vi "AutoGetRoutine.vi"(1 "Auto Routine":T6) -> (0 "Output Routine":T1[](array[typedef]))   [LabVIEW 2017]
uses:
  TypeDef/AutoRoutines.ctl
  TypeDef/AutoStep.ctl
  TypeDef/AutoWaypointType.ctl
  Pathfinder/Pathfinder-LabVIEW/Pathfinder-Lib/VIs/Waypoint.ctl
  Implements/Arm/TypeDefs/ArmTargetPosition.ctl
  Implements/TypeDefs/IntakeState.ctl
  Pathfinder/Pathfinder-LabVIEW/Pathfinder-Lib/Pathfinder.lvlib
panel:
  in  "Routines":T1[][](array[typedef])=[[{"Waypoint Type"=enum."Pathfinder Endpoint", "Waypoint"={"x"=19.5, "y"=160.0, "angle"=0.0}, "WaitTime (ms)"=0, "ArmPosition"=enum."Hold", "IntakeState"=enum."Stop", "Claw Open"=FALSE}, {"Waypoint Type"=enum."Pathfinder Endpoint", "Waypoint"={"x"=151.0, "y"=225.0, "angle"=0.0}, "WaitTime (ms)"=0, "ArmPosition"=enum."Switch", "IntakeState"=enum."Stop", "Claw Open"=FALSE}, {"Waypoint Type"=enum."Stationary", "Waypoint"={"x"=0.0, "y"=0.0, "angle"=0.0}, "WaitTime (ms)"=250, "ArmPosition"=enum."Switch", "IntakeState"=enum."Stop", "Claw Open"=TRUE}, {"Waypoint Type"=enum."Pathfinder Endpoint", "Waypoint"={"x"=0.0, "y"=0.0, "angle"=0.0}, "WaitTime (ms)"=0, "ArmPosition"=enum."Hold", "IntakeState"=enum."Stop", "Claw Open"=FALSE}, {"Waypoint Type"=enum."Pathfinder Endpoint", "Waypoint"={"x"=0.0, "y"=0.0, "angle"=0.0}, "WaitTime (ms)"=0, "ArmPosition"=enum."Hold", "IntakeState"=enum."Stop", "Claw Open"=FALSE}, {"Waypoint Type"=enum."Pathfinder Endpoint", "Waypoint"={"x"=0.0, "y"=0.0, "angle"=0.0}, "WaitTime (ms)"=0, "ArmPosition"=enum."Hold", "IntakeState"=enum."Stop", "Claw Open"=FALSE}, {"Waypoint Type"=enum."Pathfinder Endpoint", "Waypoint"={"x"=0.0, "y"=0.0, "angle"=0.0}, "WaitTime (ms)"=0, "ArmPosition"=enum."Hold", "IntakeState"=enum."Stop", "Claw Open"=FALSE}, {"Waypoint Type"=enum."Pathfinder Endpoint", "Waypoint"={"x"=0.0, "y"=0.0, "angle"=0.0}, "WaitTime (ms)"=0, "ArmPosition"=enum."Hold", "IntakeState"=enum."Stop", "Claw Open"=FALSE}, {"Waypoint Type"=enum."Pathfinder Endpoint", "Waypoint"={"x"=0.0, "y"=0.0, "angle"=0.0}, "WaitTime (ms)"=0, "ArmPosition"=enum."Hold", "IntakeState"=enum."Stop", "Claw Open"=FALSE}, {"Waypoint Type"=enum."Pathfinder Endpoint", "Waypoint"={"x"=0.0, "y"=0.0, "angle"=0.0}, "WaitTime (ms)"=0, "ArmPosition"=enum."Hold", "IntakeState"=enum."Stop", "Claw Open"=FALSE}], [{"Waypoint Type"=enum."Pathfinder Endpoint", "Waypoint"={"x"=19.5, "y"=160.0, "angle"=0.0}, "WaitTime (ms)"=0, "ArmPosition"=enum."Hold", "IntakeState"=enum."Stop", "Claw Open"=FALSE}, {"Waypoint Type"=enum."Pathfinder Endpoint", "Waypoint"={"x"=151.0, "y"=110.0, "angle"=0.0}, "WaitTime (ms)"=0, "ArmPosition"=enum."Switch", "IntakeState"=enum."Stop", "Claw Open"=FALSE}, {"Waypoint Type"=enum."Stationary", "Waypoint"={"x"=0.0, "y"=0.0, "angle"=0.0}, "WaitTime (ms)"=250, "ArmPosition"=enum."Switch", "IntakeState"=enum."Stop", "Claw Open"=TRUE}, {"Waypoint Type"=enum."Pathfinder Endpoint", "Waypoint"={"x"=0.0, "y"=0.0, "angle"=0.0}, "WaitTime (ms)"=0, "ArmPosition"=enum."Hold", "IntakeState"=enum."Stop", "Claw Open"=FALSE}, {"Waypoint Type"=enum."Pathfinder Endpoint", "Waypoint"={"x"=0.0, "y"=0.0, "angle"=0.0}, "WaitTime (ms)"=0, "ArmPosition"=enum."Hold", "IntakeState"=enum."Stop", "Claw Open"=FALSE}, {"Waypoint Type"=enum."Pathfinder Endpoint", "Waypoint"={"x"=0.0, "y"=0.0, "angle"=0.0}, "WaitTime (ms)"=0, "ArmPosition"=enum."Hold", "IntakeState"=enum."Stop", "Claw Open"=FALSE}, {"Waypoint Type"=enum."Pathfinder Endpoint", "Waypoint"={"x"=0.0, "y"=0.0, "angle"=0.0}, "WaitTime (ms)"=0, "ArmPosition"=enum."Hold", "IntakeState"=enum."Stop", "Claw Open"=FALSE}, {"Waypoint Type"=enum."Pathfinder Endpoint", "Waypoint"={"x"=0.0, "y"=0.0, "angle"=0.0}, "WaitTime (ms)"=0, "ArmPosition"=enum."Hold", "IntakeState"=enum."Stop", "Claw Open"=FALSE}, {"Waypoint Type"=enum."Pathfinder Endpoint", "Waypoint"={"x"=0.0, "y"=0.0, "angle"=0.0}, "WaitTime (ms)"=0, "ArmPosition"=enum."Hold", "IntakeState"=enum."Stop", "Claw Open"=FALSE}, {"Waypoint Type"=enum."Pathfinder Endpoint", "Waypoint"={"x"=0.0, "y"=0.0, "angle"=0.0}, "WaitTime (ms)"=0, "ArmPosition"=enum."Hold", "IntakeState"=enum."Stop", "Claw Open"=FALSE}], [{"Waypoint Type"=enum."Pathfinder Endpoint", "Waypoint"={"x"=19.5, "y"=50.0, "angle"=0.0}, "WaitTime (ms)"=0, "ArmPosition"=enum."Hold", "IntakeState"=enum."Stop", "Claw Open"=FALSE}, {"Waypoint Type"=enum."Pathfinder Endpoint", "Waypoint"={"x"=180.0, "y"=50.0, "angle"=0.0}, "WaitTime (ms)"=0, "ArmPosition"=enum."Hold", "IntakeState"=enum."Stop", "Claw Open"=FALSE}, {"Waypoint Type"=enum."Zero-Radius Turn Endpoint", "Waypoint"={"x"=0.0, "y"=0.0, "angle"=0.0}, "WaitTime (ms)"=0, "ArmPosition"=enum."Hold", "IntakeState"=enum."Stop", "Claw Open"=FALSE}, {"Waypoint Type"=enum."Zero-Radius Turn Endpoint", "Waypoint"={"x"=0.0, "y"=0.0, "angle"=110.0}, "WaitTime (ms)"=0, "ArmPosition"=enum."Switch", "IntakeState"=enum."Stop", "Claw Open"=FALSE}, {"Waypoint Type"=enum."Pathfinder Endpoint", "Waypoint"={"x"=180.0, "y"=50.0, "angle"=90.0}, "WaitTime (ms)"=0, "ArmPosition"=enum."Switch", "IntakeState"=enum."Stop", "Claw Open"=FALSE}, {"Waypoint Type"=enum."Pathfinder Endpoint", "Waypoint"={"x"=180.0, "y"=80.0, "angle"=90.0}, "WaitTime (ms)"=0, "ArmPosition"=enum."Switch", "IntakeState"=enum."Stop", "Claw Open"=FALSE}, {"Waypoint Type"=enum."Stationary", "Waypoint"={"x"=0.0, "y"=0.0, "angle"=0.0}, "WaitTime (ms)"=250, "ArmPosition"=enum."Switch", "IntakeState"=enum."Stop", "Claw Open"=TRUE}, {"Waypoint Type"=enum."Pathfinder Endpoint", "Waypoint"={"x"=0.0, "y"=0.0, "angle"=0.0}, "WaitTime (ms)"=0, "ArmPosition"=enum."Hold", "IntakeState"=enum."Stop", "Claw Open"=FALSE}, {"Waypoint Type"=enum."Pathfinder Endpoint", "Waypoint"={"x"=0.0, "y"=0.0, "angle"=0.0}, "WaitTime (ms)"=0, "ArmPosition"=enum."Hold", "IntakeState"=enum."Stop", "Claw Open"=FALSE}, {"Waypoint Type"=enum."Pathfinder Endpoint", "Waypoint"={"x"=0.0, "y"=0.0, "angle"=0.0}, "WaitTime (ms)"=0, "ArmPosition"=enum."Hold", "IntakeState"=enum."Stop", "Claw Open"=FALSE}], [{"Waypoint Type"=enum."Pathfinder Endpoint", "Waypoint"={"x"=19.5, "y"=50.0, "angle"=0.0}, "WaitTime (ms)"=0, "ArmPosition"=enum."Hold", "IntakeState"=enum."Stop", "Claw Open"=FALSE}, {"Waypoint Type"=enum."Pathfinder Waypoint", "Waypoint"={"x"=180.0, "y"=50.0, "angle"=0.0}, "WaitTime (ms)"=0, "ArmPosition"=enum."Hold", "IntakeState"=enum."Stop", "Claw Open"=FALSE}, {"Waypoint Type"=enum."Pathfinder Waypoint", "Waypoint"={"x"=270.0, "y"=135.0, "angle"=90.0}, "WaitTime (ms)"=0, "ArmPosition"=enum."Hold", "IntakeState"=enum."Stop", "Claw Open"=FALSE}, {"Waypoint Type"=enum."Pathfinder Waypoint", "Waypoint"={"x"=270.0, "y"=260.0, "angle"=90.0}, "WaitTime (ms)"=0, "ArmPosition"=enum."Hold", "IntakeState"=enum."Stop", "Claw Open"=FALSE}, {"Waypoint Type"=enum."Pathfinder Endpoint", "Waypoint"={"x"=180.0, "y"=350.0, "angle"=180.0}, "WaitTime (ms)"=0, "ArmPosition"=enum."Hold", "IntakeState"=enum."Stop", "Claw Open"=FALSE}, {"Waypoint Type"=enum."Zero-Radius Turn Endpoint", "Waypoint"={"x"=0.0, "y"=0.0, "angle"=180.0}, "WaitTime (ms)"=0, "ArmPosition"=enum."Hold", "IntakeState"=enum."Stop", "Claw Open"=FALSE}, {"Waypoint Type"=enum."Zero-Radius Turn Endpoint", "Waypoint"={"x"=0.0, "y"=0.0, "angle"=290.0}, "WaitTime (ms)"=0, "ArmPosition"=enum."Switch", "IntakeState"=enum."Stop", "Claw Open"=FALSE}, {"Waypoint Type"=enum."Pathfinder Endpoint", "Waypoint"={"x"=180.0, "y"=320.0, "angle"=270.0}, "WaitTime (ms)"=0, "ArmPosition"=enum."Switch", "IntakeState"=enum."Stop", "Claw Open"=FALSE}, {"Waypoint Type"=enum."Pathfinder Endpoint", "Waypoint"={"x"=180.0, "y"=300.0, "angle"=270.0}, "WaitTime (ms)"=0, "ArmPosition"=enum."Switch", "IntakeState"=enum."Stop", "Claw Open"=FALSE}, {"Waypoint Type"=enum."Stationary", "Waypoint"={"x"=0.0, "y"=0.0, "angle"=0.0}, "WaitTime (ms)"=250, "ArmPosition"=enum."Switch", "IntakeState"=enum."Stop", "Claw Open"=TRUE}]]
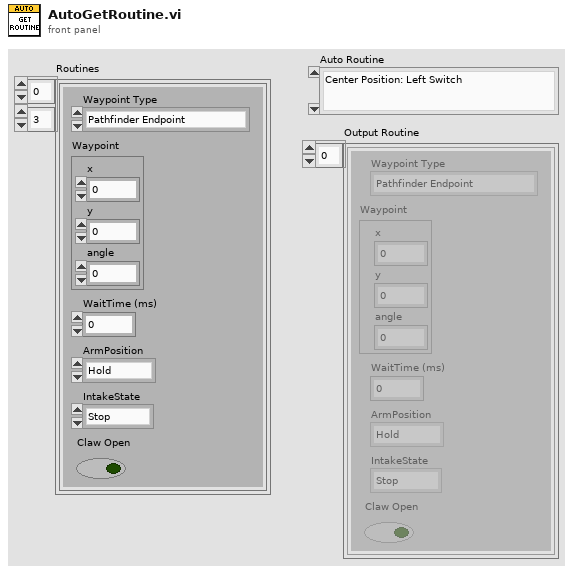
[diagram p1: front panel]
types:
  T1 = typedef "AutoStep.ctl" = cluster{"Waypoint Type":T2, "Waypoint":T3, "WaitTime (ms)":u16, "ArmPosition":T4, "IntakeState":T5, "Claw Open":bool}
  T2 = typedef "AutoWaypointType.ctl" = enum16{"Pathfinder Endpoint", "Pathfinder Waypoint", "Zero-Radius Turn Endpoint", "Stationary", "Vision Assist Endpoint"}
  T3 = typedef "Pathfinder.lvlib/Waypoint.ctl" = cluster{"x":dbl, "y":dbl, "angle":dbl}
  T4 = typedef "ArmTargetPosition.ctl" = enum16{"Hold", "Switch", "Scale Low", "Scale High", "Climb"}
  T5 = typedef "IntakeState.ctl" = enum16{"Stop", "Forward", "Reverse", "Forward Open"}
  T6 = typedef "AutoRoutines.ctl" = enum16{"Center Position: Left Switch", "Center Position: Right Switch", "Right Position: Right Switch", "Right Position: Left Switch"}
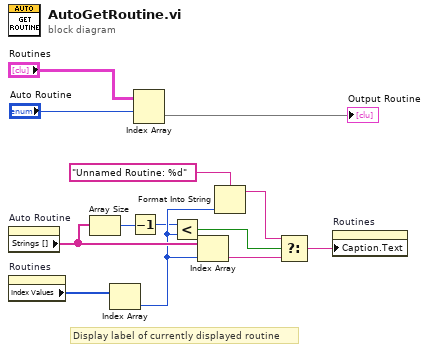
[diagram p0: block diagram]
diagram:
  # "Display label of currently displayed routine"
  n1 = property on="Auto Routine" class="Enum (strict)"() -> ("Strings []"=w9:string[])  [unwired: 2 in, 2 out]
  n2 = property on="Routines" class="Arr (strict)"() -> ("Index Values"=w10:u32[])  [unwired: 2 in, 2 out]
  n3 = Array Size(array=w9) -> (size(s)=w8:i32)
  n4 = Index Array(array=w10) -> (element=w3:u32)  [unwired: 1 in]
  n5 = Decrement(x=w8) -> (x-1=w1:i32)
  n6 = Index Array(array="Routines", index (row)="Auto Routine") -> (element=→"Output Routine":T1[])  [unwired: 1 in]
  n7 = Less?(x=w1, y=w3) -> (x < y?=w5:bool)
  n8 = Index Array(array=w9, index=w3) -> (element=w7:string)
  n9 = Format Into String(format string="Unnamed Routine: %d" ("t"), w3) -> (resulting string=w2:string)  [unwired: 2 in, 1 out]
  n10 = Select(t=w2, s=w5, f=w7) -> (s? t:f=w6:string)
  n11 = property on="Routines" class="Arr (strict)"("Caption.Text"=w6) -> ()  [unwired: 2 in, 2 out]
